vi "Configure.vi"(8 "error in (no error)":errorcluster, 9 "Term Char":string, 10 "VISA":refnum<visa-resource-name>) -> (0 "error out":errorcluster, 3 "Serial out":refnum<class "Serial.lvclass">)   [LabVIEW 2021, in "Communication.lvlib" / "Serial.lvclass"]
uses:
  Serial.lvclass
  Serial.lvclass/Serial.ctl
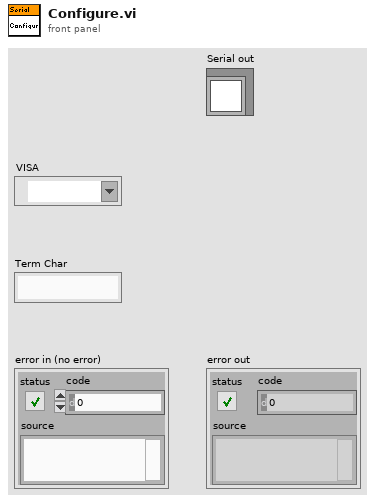
[diagram p1: front panel]
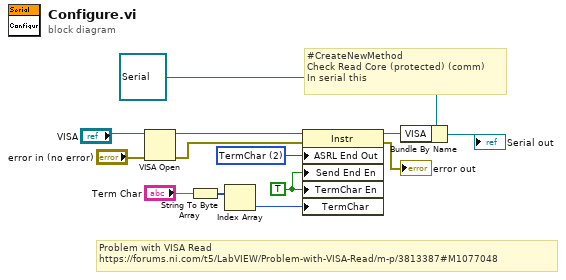
[diagram p0: block diagram]
diagram:
  w2 = u16 2 items=["None", "Last Bit", "TermChar", "Break"] ("Serial Settings:End Mode for Writes")
  w3 = TRUE ("Message Based Settings:Termination Character Enable")
  # "Problem with VISA Read\nhttps://forums.ni.com/t5/LabVIEW/Problem-with-VISA-Read/m-p/3813387#M1077048"
  # "#CreateNewMethod\nCheck Read Core (protected) (comm)\nIn serial this"
  n1 = VISA Open(error in (no error)="error in (no error)", VISA resource name="VISA") -> (VISA resource name=w10:refnum<visa-resource-name>, error out=w7:errorcluster)  [unwired: 3 in]
  n2 = String To Byte Array(string="Term Char") -> (unsigned byte array=w8:u8[])
  n3 = Index Array(array=w8) -> (element=w6:u8)  [unwired: 1 in]
  n4 = property class="Instr"(reference=w10, error in=w7, "ASRL End Out"=w2, "Send End En"=w3, "TermChar En"=w3, "TermChar"=w6) -> (reference out=w9:refnum<visa-resource-name>, error out=→"error out":errorcluster)
  n5 = Bundle By Name(cluster=refnum<class "Serial.lvclass"> refnum ("Serial in"), "VISA"=w9) -> (→"Serial out":refnum<class "Serial.lvclass">)
